vi "Get ErrorRemote Event.vi"(8 "error in (no error)":errorcluster, 11 "ErrorHandler in":refnum<class "ErrorHandler.lvclass">) -> (0 "error out":errorcluster, 2 "ErrorRemote Ev":refnum<user-event>, 3 "ErrorHandler out":refnum<class "ErrorHandler.lvclass">)   [LabVIEW 2019, in "ErrorHandler.lvclass"]
doc: "Developed by Kevin Thompson\nkevin@thompsonengineering.net\n\nCopyright 2018\nThompson Engineering, LLC"
uses:
  ErrorHandler.lvclass
  TypeDef/ErrorRemote EventData.ctl
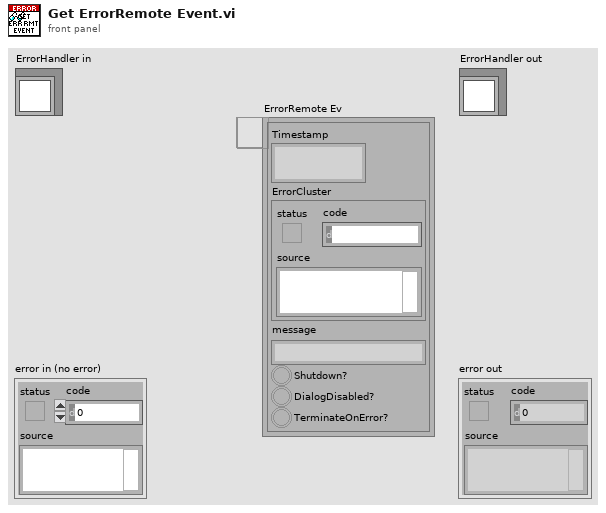
[diagram p1: front panel]
types:
  T1 = typedef "ErrorHandler.lvclass/ObjData--cluster.ctl" = cluster{"AppName":string, "ErrorLogBasePath":path, "ErrorDialogPopUp Disabled":bool, "TerminateAppOnError Enabled":bool, "Public Events":T2, "ErrorList Qref":refnum<queue>}
  T2 = typedef "ErrorHandler.lvclass/Public Events.ctl" = cluster{"ErrorRemote Ev":refnum<user-event>}
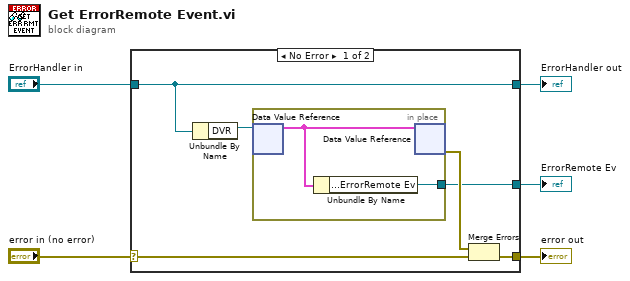
[diagram p0: block diagram]
diagram:
  n1 = case shown="No Error" "error in (no error)" {
    selector: "error in (no error)" -> [w6 w14]
    tunnel: [w7 w14] -> w4
    tunnel: [w9 w15] -> w2
    tunnel: "ErrorHandler in" -> [w9 w15]
    tunnel: [w8 _] -> w1
    frame No Error {
      n2 = Unbundle By Name(w9) -> ("DVR"=w11:refnum<data-value>)
      n3 = in-place {
        in-place-border: [w13] -> w8
        n4 = in-place-dvr #1(w11) -> (w12:T1)  [unwired: 1 out]
        n5 = Unbundle By Name(w12) -> ("Public Events.ErrorRemote Ev"=w13:refnum<user-event>)
        n6 = in-place-dvr #1(w12) -> (w10:errorcluster)  [unwired: 1 out]
      }
      n7 = Merge Errors(w10, w6) -> (w7:errorcluster)
    }
    frame Error {
    }
  }
  "error out" <- w4
  "ErrorHandler out" <- w2
  "ErrorRemote Ev" <- w1
